vi "Example_Write.vi"() -> ()   [LabVIEW 2021]
panel:
  out "output waveform":waveform(i32)
  in  "file path (use dialog)":path
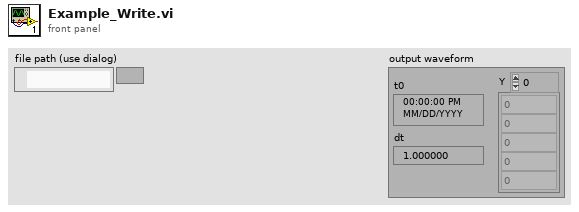
[diagram p1: front panel]
types:
  T1 = enum16{"open", "replace", "create", "open or create", "replace or create", "replace or create with confirmation"}
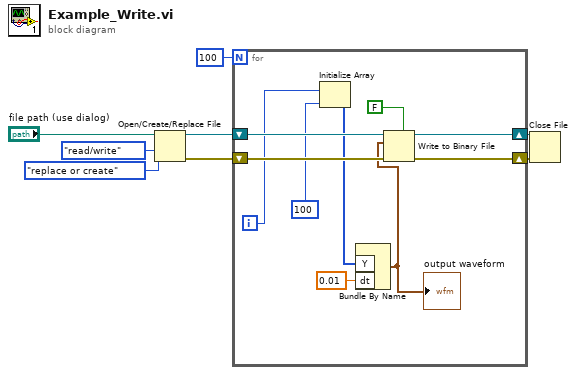
[diagram p0: block diagram]
diagram:
  n1 = Open/Create/Replace File(file path (use dialog)="file path (use dialog)", operation (0:open)=T1."replace or create", access (0:read/write)=enum16{"read/write", "read-only", "write-only"}."read/write") -> (refnum out=w8:refnum<file>, error out=w7:errorcluster)  [unwired: 3 in, 1 out]
  n2 = for {
    N: 100 -> [_]
    shift-right: [w16] -> w6
    shift-left: w8 -> [w18]
    shift-right: [w15] -> w5
    shift-left: w7 -> [w17]
    i -> [w14]
    n3 = Initialize Array(w14, 100 ("element")) -> (w11:i32[])
    n4 = Bundle By Name("Y"=w11, "dt"=0.01) -> (w9:waveform(i32))  [unwired: 1 in]
    "output waveform" <- w9
    n5 = Write to Binary File(file (use dialog)=w18, data=w9, error in=w17, 5:FALSE ("prepend array or string size? (T)")) -> (refnum out=w16:refnum<file>, error out=w15:errorcluster)  [unwired: 2 in, 1 out]
  }
  n6 = Close File(refnum=w6, error in=w5) -> ()  [unwired: 2 out]
